vi "Pre Proceed Image.vi"(8 "error in (no error)":errorcluster, 11 "HIJ IMAQdx Display in":refnum<class "HIJ IMAQdx Display.lvclass">) -> (0 "error out":errorcluster, 3 "HIJ IMAQdx Display out":refnum<class "HIJ IMAQdx Display.lvclass">)   [LabVIEW 2014, in "HIJ IMAQdx Display.lvlib" / "HIJ IMAQdx Display.lvclass"]
uses:
  HIJ IMAQdx Display.lvclass
  HIJ IMAQdx Display.lvclass/HIJ IMAQdx Display.ctl
  HIJ Vision Display/HIJ Vision Display/HIJ Vision Display.lvclass/HIJ Vision Display.ctl
  HIJ Vision Display/HIJ Vision Display/Read Display Image 2.vi
  HIJ Vision Display/HIJ Vision Display/HIJ Vision Display.lvclass
  <vilib>/vision/NI_Vision_Development_Module.lvlib
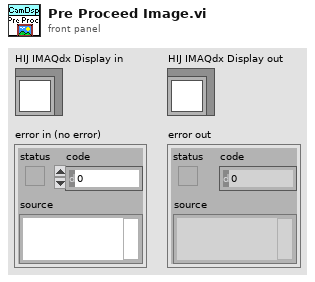
[diagram p1: front panel]
types:
  T1 = typedef "IMAQ Image.ctl" = refnum<image>
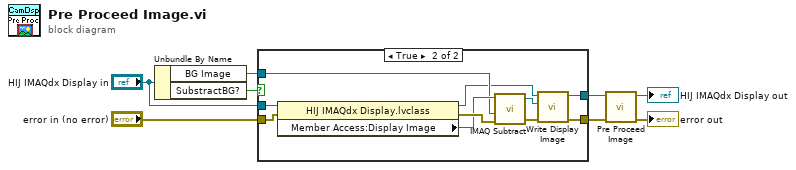
[diagram p0: block diagram]
diagram:
  n1 = Unbundle By Name("HIJ IMAQdx Display in") -> ("BG Image"=w7:T1, "SubstractBG?"=w1:bool)
  n2 = case shown="True" w1 {
    tunnel: w7 -> [_ w16]
    tunnel: "error in (no error)" -> [w10 w19]
    tunnel: [w10 w11] -> w5
    tunnel: "HIJ IMAQdx Display in" -> [w9 w20]
    tunnel: [w9 w14] -> w2
    frame False {
    }
    frame True {
      n3 = property class="HIJ IMAQdx Display.lvclass"(reference=w20, error in=w19) -> (reference out=w15:refnum<class "HIJ IMAQdx Display.lvclass">, error out=w18:errorcluster, "Member Access:Display Image"=w17:T1)
      n4 = call "IMAQ Subtract"("Image Src A"=w17, "Image Src B"=w16, "error in (no error)"=w18) -> ("Image Dst Out"=w13:T1, "error out"=w12:errorcluster)  [unwired: 4 in]
      n5 = call "Write Display Image.vi"("error in (no error)"=w12, "Image"=w13, "HIJ Vision Display in"=w15) -> ("error out"=w11:errorcluster, "HIJ Vision Display out"=w14:refnum<class "HIJ IMAQdx Display.lvclass">)  [unwired: 7 in]
    }
  }
  n6 = call-parent "Pre Proceed Image.vi"("error in (no error)"=w5, "Display in"=w2) -> ("error out"=→"error out":errorcluster, "Display out"=→"HIJ IMAQdx Display out":refnum<class "HIJ IMAQdx Display.lvclass">)  [unwired: 8 in]
